vi "maybe obsolete.vi"(8 "error in (no error)":errorcluster, 9 "Value":string, 10 "Ring Refnum":refnum<vi>, 11 "MulticolumnListbox in":refnum<vi>) -> (3 "Array":i32[](array[numeric]))   [LabVIEW 2020]
uses:
  <userlib>/_OpenG.lib/array/array.llb/Sort 2D Array (String)__ogtk.vi
  <userlib>/_OpenG.lib/array/array.llb/openg_array.lvlib
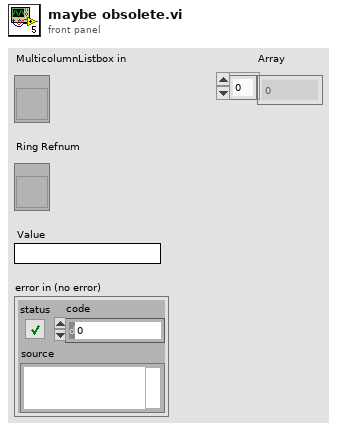
[diagram p1: front panel]
types:
  T1 = typedef "mysql_authentication.ctl" = cluster{"User":string, "Password":string, "Database":string}
  T2 = cluster{"Port":u16, "IP Address":string, "Authentication":T1}
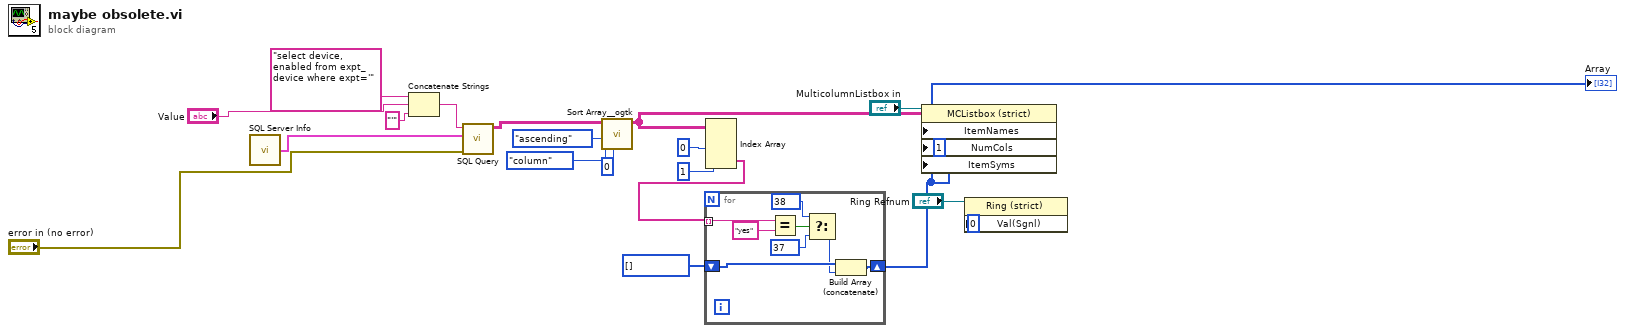
[diagram p0: block diagram]
diagram:
  n1 = call "SQL Server Info.vi"() -> ("SQL Server Info"=w7:T2)
  n2 = Concatenate Strings("select device, enabled from expt_device where expt='" ("Query"), "Value", "'" ("Query")) -> (w3:string)
  n3 = call "SQL Query.vi"("error in (no error)"="error in (no error)", "SQL Server Info"=w7, "Query"=w3) -> ("data"=w14:string[][])  [unwired: 7 in, 1 out]
  n4 = call-poly <userlib>:"Sort Array__ogtk.vi"("Column/Row to Sort By"=u32 0, "Sort By in"=enum16{"row", "column"}."column", "Order"=enum16{"ascending", "descending"}."ascending", "Array in"=w14) -> ("Sorted Array out"=w18:string[][])  [unwired: 4 in, 3 out]
  n5 = Index Array(array=w18, index (col) #1=0 ("disabled index (col)"), index (col) #2=1 ("index (col)")) -> (element #2=w11:string[])  [unwired: 2 in, 1 out]
  n6 = for {
    tunnel: w11 -> [w28] mode=indexing
    shift-right: [w21] -> w13
    shift-left: i32[] [] -> [w26]
    n7 = Equal?(x=w28, y="yes") -> (x = y?=w25:bool)
    n8 = Select(t=38, s=w25, f=37) -> (s? t:f=w22:i32)
    n9 = Build Array (concatenate)(w26, w22) -> (w21:i32[])
  }
  "Array" <- w13
  n10 = property on="Property Node" class="MCListbox (strict)"(reference="MulticolumnListbox in", "ItemNames"=w18, "NumCols"=u32 1 ("Number of Columns"), "ItemSyms"=w13) -> ()  [unwired: 1 in, 2 out]
  n11 = property on="Property Node" class="Ring (strict)"(reference="Ring Refnum", "Val(Sgnl)"=u16 0 ("Value (Signaling)")) -> ()  [unwired: 1 in, 2 out]
